vi "Measure_FUN_Read value.vi"(7 "Read Action":enum16{"Initialize", "Read Value", "Read State"}(ring), 8 "Error In":errorcluster, 11 "VISA In":refnum<visa-resource-name>) -> (0 "Error Out":errorcluster, 1 "Value":dbl, 2 "State":T1, 3 "VISA Out":refnum<visa-resource-name>)   [LabVIEW 2015]
panel:
  out "return count":u32
  in  "Time out":u32=3000
  out "Mode(Number)":i32
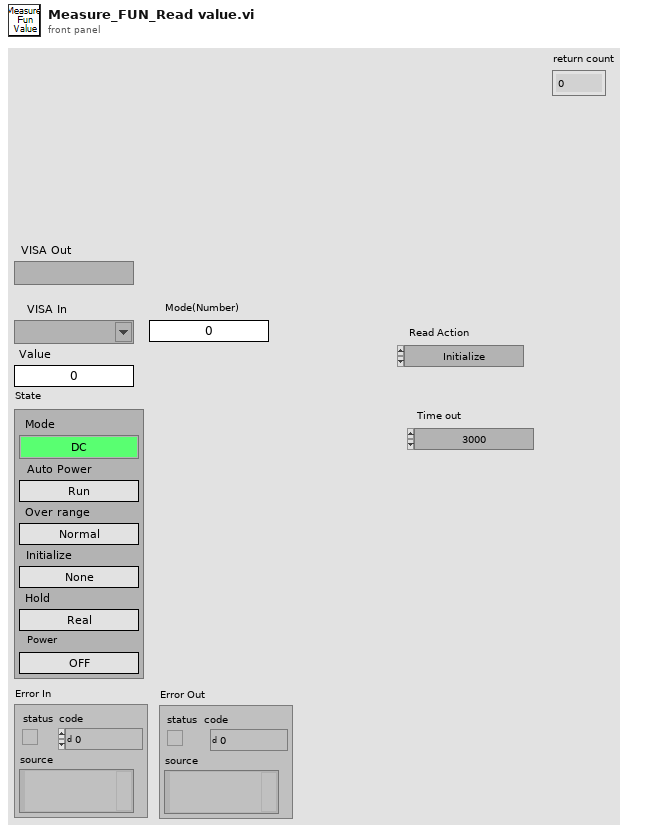
[diagram p1: front panel]
types:
  T1 = cluster{"Mode":enum16{"DC", "DC*10", "AC*10"}, "Auto Power":bool, "Over range":bool, "Initialize":bool, "Hold":bool, "Power":bool}
  T2 = cluster{"Mode":enum16{"DC", "DC*10", "AC*10"}, bool, bool, bool, bool, bool}
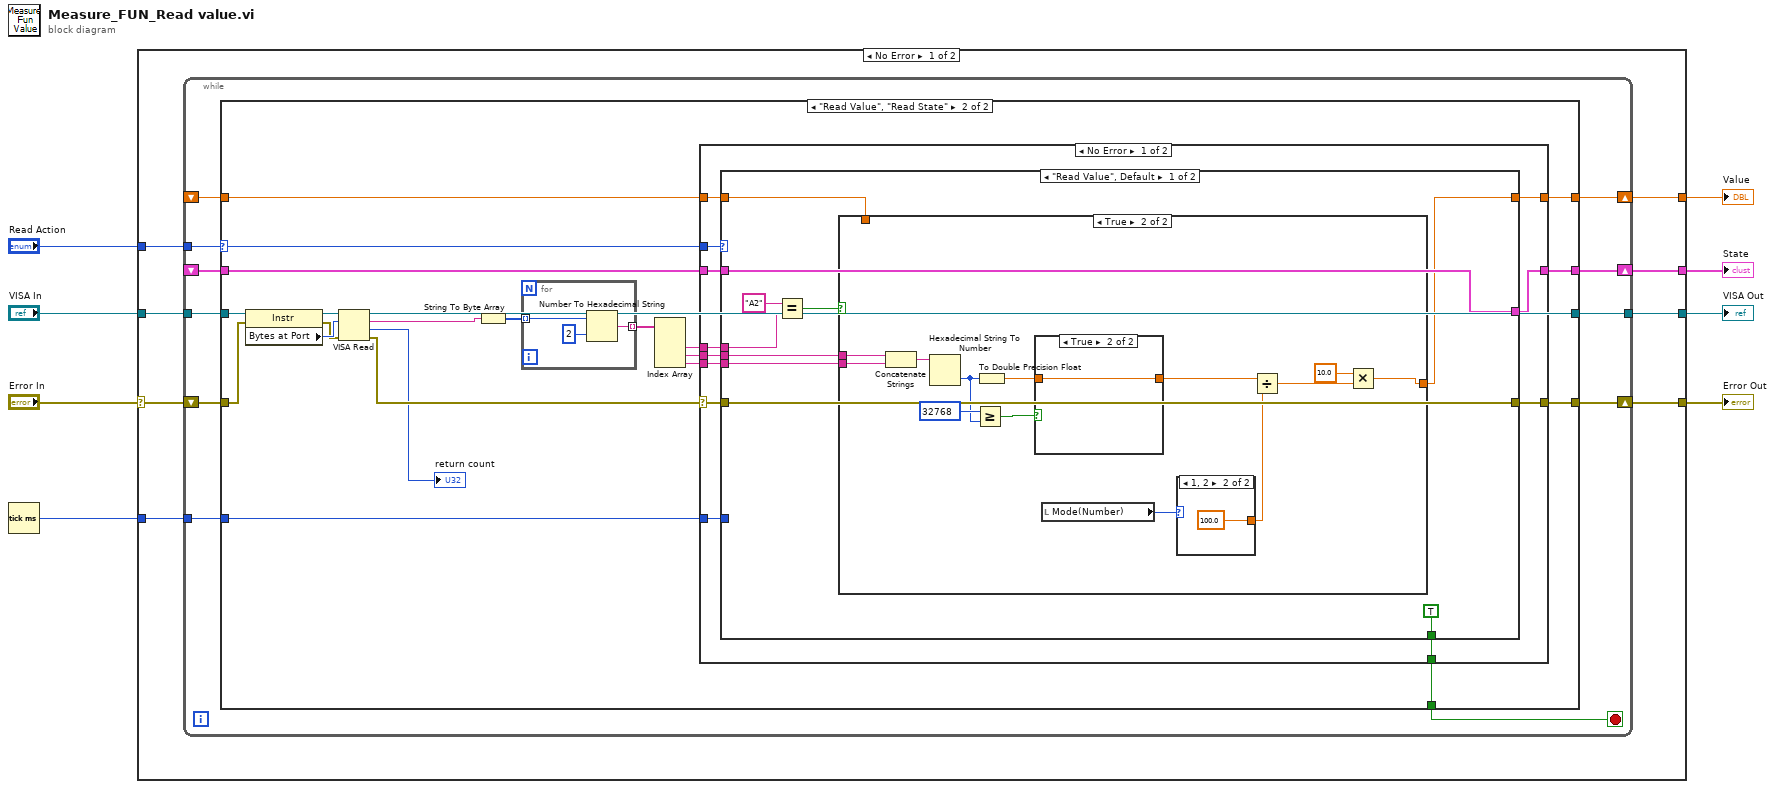
[diagram p0: block diagram]
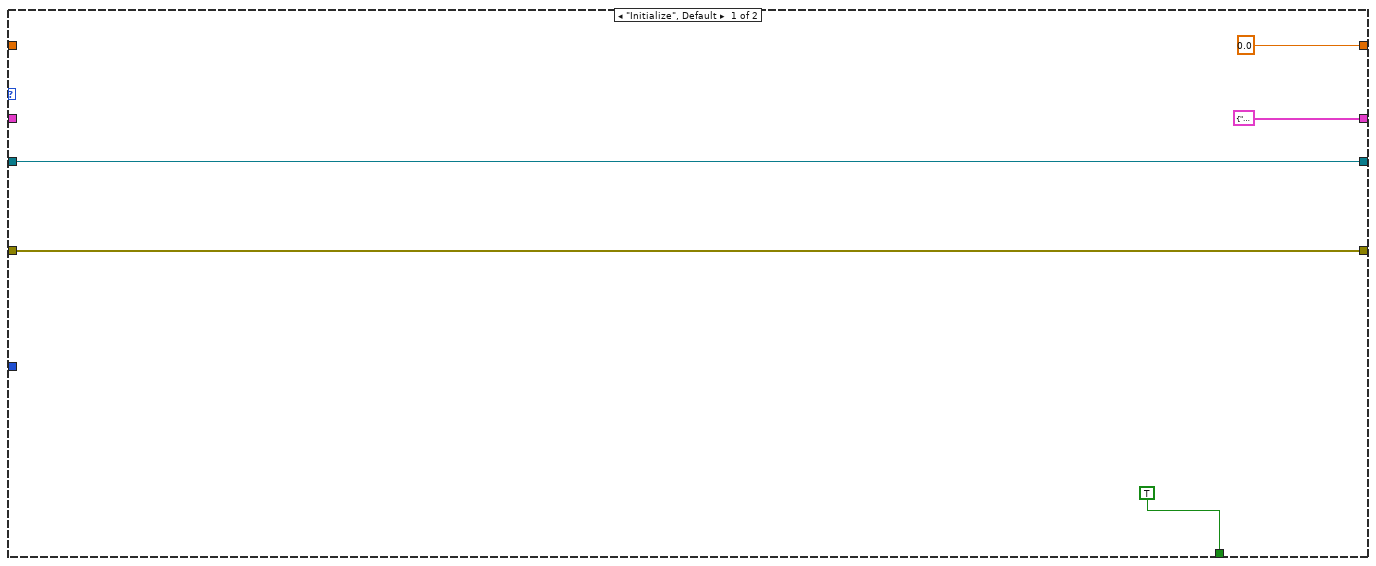
[diagram p2: hidden frame]
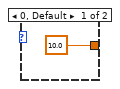
[diagram p4: hidden frame]
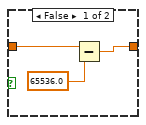
[diagram p5: hidden frame]
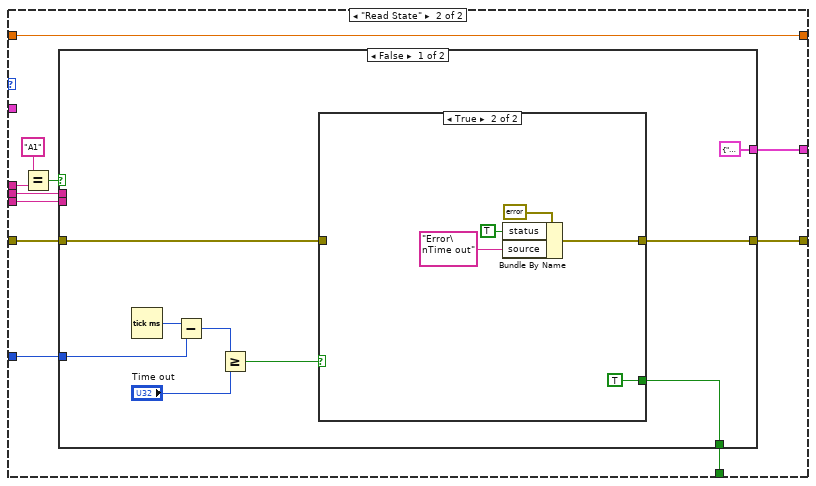
[diagram p6: hidden frame]
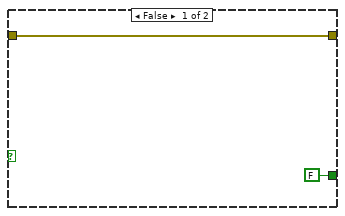
[diagram p7: hidden frame]
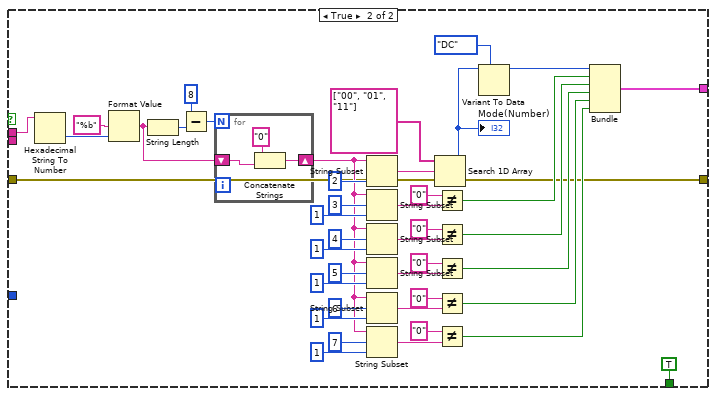
[diagram p8: hidden frame]
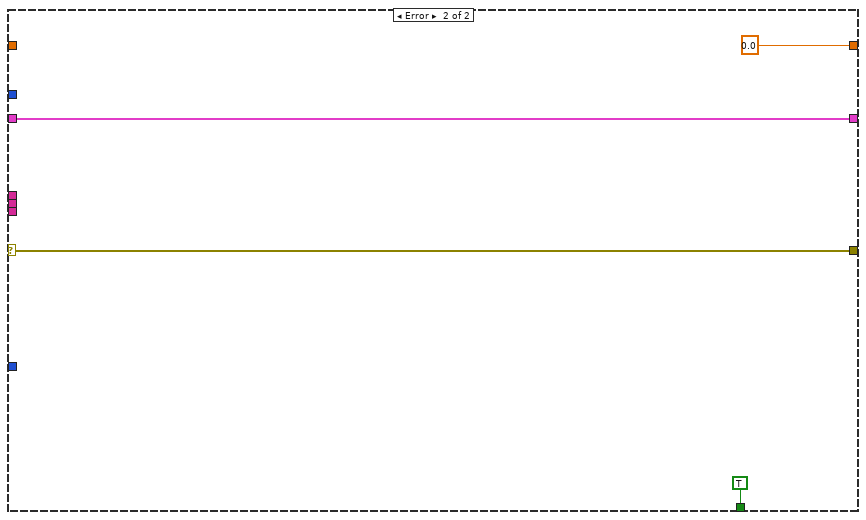
[diagram p9: hidden frame]
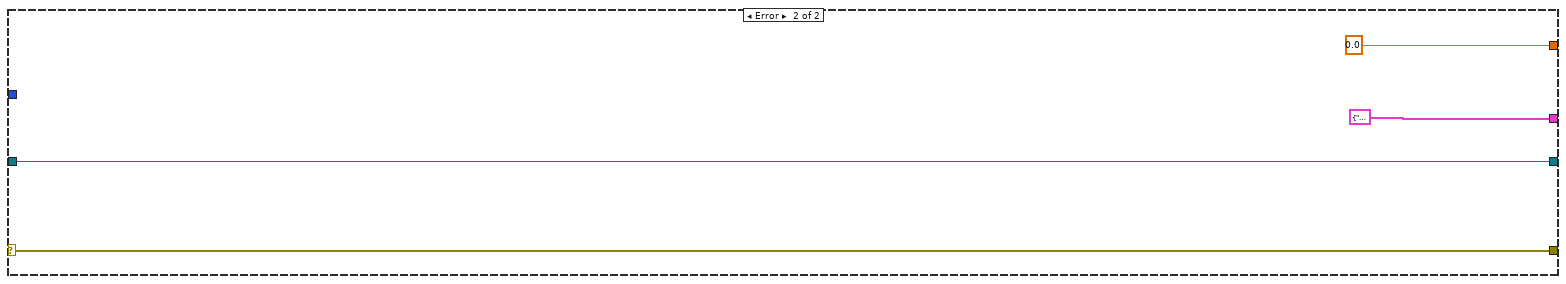
[diagram p10: hidden frame]
diagram:
  n1 = Tick Count (ms)() -> (millisecond timer value=w4:u32)
  n2 = case shown="No Error" "Error In" {
    selector: "Error In" -> [w15 w179]
    tunnel: "VISA In" -> [w16 w178]
    tunnel: [w14 w179] -> w6
    tunnel: "Read Action" -> [w13 _]
    tunnel: w4 -> [w12 _]
    tunnel: [w11 w178] -> w3
    tunnel: [w10 0.0] -> w2
    tunnel: [w9 T1 {"Mode"=enum."DC", "Auto Power"=FALSE, "Over range"=FALSE, "Initialize"=FALSE, "Hold"=FALSE, "Power"=FALSE} ("State")] -> w1
    frame No Error {
      n3 = while {
        tunnel: w16 -> [w27]
        shift-right: [w23] -> w14
        shift-left: w15 -> [w26]
        tunnel: w13 -> [w19]
        tunnel: w12 -> [w24]
        tunnel: [w22] -> w11
        shift-right: [w21] -> w10
        shift-left: _ -> [w20]
        shift-right: [w18] -> w9
        shift-left: _ -> [w17]
        stop <- w25 stop-if-true
        n4 = case shown="\"Read Value\", \"Read State\"" w19 {
          selector: w19 -> [_ w41]
          tunnel: w27 -> [w31 w54]
          tunnel: w26 -> [w30 w49]
          tunnel: [TRUE w48] -> w25
          tunnel: w24 -> [_ w47]
          tunnel: [w30 w46] -> w23
          tunnel: [w31 w44] -> w22
          tunnel: [0.0 w43] -> w21
          tunnel: w20 -> [_ w42]
          tunnel: [T1 {"Mode"=enum."DC", "Auto Power"=FALSE, "Over range"=FALSE, "Initialize"=FALSE, "Hold"=FALSE, "Power"=FALSE} ("State") w40] -> w18
          tunnel: w17 -> [_ w39]
          frame "Initialize", Default {
          }
          frame "Read Value", "Read State" {
            n5 = property class="Instr"(reference=w54, error in=w49) -> (reference out=w52:refnum<visa-resource-name>, error out=w51:errorcluster, "Bytes at Port"=w53:u32)
            n6 = VISA Read(VISA resource name=w52, byte count=w53, error in (no error)=w51) -> (VISA resource name out=w44:refnum<visa-resource-name>, read buffer=w50:string, return count=→"return count":u32, error out=w45:errorcluster)
            n7 = String To Byte Array(string=w50) -> (unsigned byte array=w38:u8[])
            n8 = for {
              tunnel: w38 -> [w55] mode=indexing
              tunnel: [w57] -> w37 mode=indexing
              n9 = Number To Hexadecimal String(1:i16 2 ("width (-)"), 2:w55) -> (0:w57:string)
            }
            n10 = Index Array(array=w37) -> (element #2=w34:string, element #3=w36:string, element #4=w35:string)  [unwired: 4 in, 1 out]
            n11 = case shown="No Error" w45 {
              selector: w45 -> [w62 w175]
              tunnel: w36 -> [w69 _]
              tunnel: w35 -> [w68 _]
              tunnel: w34 -> [w67 _]
              tunnel: [w66 TRUE] -> w48
              tunnel: w41 -> [w65 _]
              tunnel: w47 -> [w64 _]
              tunnel: [w63 w175] -> w46
              tunnel: [w61 0.0] -> w43
              tunnel: w42 -> [w60 _]
              tunnel: [w59 w172] -> w40
              tunnel: w39 -> [w58 w172]
              frame No Error {
                n12 = case shown="\"Read Value\", Default" w65 {
                  tunnel: w69 -> [w79 w107]
                  tunnel: w68 -> [w78 w106]
                  tunnel: w67 -> [w74 w109]
                  tunnel: [TRUE w105] -> w66
                  tunnel: w64 -> [_ w104]
                  tunnel: [w76 w103] -> w63
                  tunnel: w62 -> [w76 w102]
                  tunnel: [w70 w101] -> w61
                  tunnel: w60 -> [w72 w101]
                  tunnel: [w71 w100] -> w59
                  tunnel: w58 -> [w71 _]
                  frame "Read Value", Default {
                    n13 = Equal?(x="A2", y=w74) -> (x = y?=w75:bool)
                    n14 = case shown="True" w75 {
                      tunnel: w79 -> [_ w93]
                      tunnel: w78 -> [_ w92]
                      tunnel: [w80 w81] -> w70
                      tunnel: w72 -> [w80 _]
                      frame False {
                      }
                      frame True {
                        n15 = Concatenate Strings(w93, w92) -> (w91:string)
                        n16 = Hexadecimal String To Number(string=w91) -> (number=w89:u32)  [unwired: 2 in, 1 out]
                        n17 = Greater Or Equal?(x=u32 32768, y=w89) -> (x >= y?=w87:bool)
                        n18 = To Double Precision Float(number=w89) -> (double precision float=w88:dbl)
                        n19 = case shown="True" w87 {
                          tunnel: w88 -> [w97 w99]
                          tunnel: [w98 w99] -> w86
                          frame False {
                            n20 = Subtract(x=w97, y=65536.0) -> (x-y=w98:dbl)
                          }
                          frame True {
                          }
                        }
                        n21 = local read "Mode(Number)"() -> (w85:i32)
                        n22 = case shown="1, 2" w85 {
                          tunnel: [10.0 ("y") 100.0 ("y")] -> w84
                          frame 0, Default {
                          }
                          frame 1, 2 {
                          }
                        }
                        n23 = Divide(x=w86, y=w84) -> (x/y=w82:dbl)
                        n24 = Multiply(x=10.0, y=w82) -> (x*y=w81:dbl)
                      }
                    }
                  }
                  frame "Read State" {
                    n25 = Equal?(x="A1", y=w109) -> (x = y?=w108:bool)
                    n26 = case shown="False" w108 {
                      tunnel: w107 -> [_ w167]
                      tunnel: w106 -> [_ _]
                      tunnel: [w113 TRUE] -> w105
                      tunnel: w104 -> [w118 _]
                      tunnel: [w114 w131] -> w103
                      tunnel: w102 -> [w112 w131]
                      tunnel: [T2 {"Mode"=enum."DC", FALSE, FALSE, FALSE, FALSE, FALSE} w127] -> w100
                      frame False {
                        n27 = Tick Count (ms)() -> (millisecond timer value=w119:u32)
                        n28 = Subtract(x=w119, y=w118) -> (x-y=w117:u32)
                        n29 = Greater Or Equal?(x=w117, y="Time out") -> (x >= y?=w115:bool)
                        n30 = case shown="True" w115 {
                          tunnel: [w120 w125] -> w114
                          tunnel: [FALSE TRUE] -> w113
                          tunnel: w112 -> [w120 _]
                          frame False {
                          }
                          frame True {
                            n31 = Bundle By Name(cluster=errorcluster {"status"=FALSE, "code"=0, "source"=""} ("error out"), "status"=TRUE, "source"="Error\nTime out") -> (w125:errorcluster)
                          }
                        }
                      }
                      frame True {
                        n32 = Hexadecimal String To Number(string=w167) -> (number=w166:u32)  [unwired: 2 in, 1 out]
                        n33 = Format Value(format string="%b", value (0)=w166) -> (output string=w163:string)  [unwired: 1 in]
                        n34 = String Length(string=w163) -> (length=w164:i32)
                        n35 = Subtract(x=8, y=w164) -> (x-y=w162:i32)
                        n36 = for {
                          N: w162 -> [_]
                          shift-right: [w171] -> w150
                          shift-left: w163 -> [w169]
                          n37 = Concatenate Strings("0" ("string"), w169) -> (w171:string)
                        }
                        n38 = String Subset(string=w150, length (rest)=2 ("length (rest)")) -> (substring=w139:string)  [unwired: 1 in]
                        n39 = String Subset(string=w150, offset (0)=3, length (rest)=1 ("length (rest)")) -> (substring=w148:string)
                        n40 = String Subset(string=w150, offset (0)=4, length (rest)=1 ("length (rest)")) -> (substring=w146:string)
                        n41 = String Subset(string=w150, offset (0)=5, length (rest)=1 ("length (rest)")) -> (substring=w144:string)
                        n42 = String Subset(string=w150, offset (0)=6, length (rest)=1 ("length (rest)")) -> (substring=w142:string)
                        n43 = String Subset(string=w150, offset (0)=7, length (rest)=1 ("length (rest)")) -> (substring=w140:string)
                        n44 = Search 1D Array(1D array=string[] ["00", "01", "11"], element=w139) -> (index of element=w128:i32)  [unwired: 1 in]
                        "Mode(Number)" <- w128
                        n45 = Not Equal?(x="0", y=w148) -> (x != y?=w137:bool)
                        n46 = Not Equal?(x="0", y=w146) -> (x != y?=w136:bool)
                        n47 = Not Equal?(x="0", y=w144) -> (x != y?=w135:bool)
                        n48 = Not Equal?(x="0", y=w142) -> (x != y?=w134:bool)
                        n49 = Not Equal?(x="0", y=w140) -> (x != y?=w133:bool)
                        n50 = Variant To Data(type=enum16{"DC", "DC*10", "AC*10"}."DC" ("Mode"), Variant=w128) -> (data=w129:enum16{"DC", "DC*10", "AC*10"})  [unwired: 1 in, 1 out]
                        n51 = Bundle("Mode"=w129, w137, w136, w135, w134, w133) -> (w127:T2)  [unwired: 1 in]
                      }
                    }
                  }
                }
              }
              frame Error {
              }
            }
          }
        }
      }
    }
    frame Error {
    }
  }
  "Error Out" <- w6
  "VISA Out" <- w3
  "Value" <- w2
  "State" <- w1
